vi "RamCtrl_Traj_UpdDiagGlobals.vi"(9 "outRAMSETE (SI)":T1 {"poseError"."ROTATION"."SIN" format="%13.4f"; "poseError"."ROTATION"."COS" format="%13.4f"; "poseError"."ROTATION"."VALUE" format="%13.4f"; "poseError"."TRANSLATION"."Y" format="%14.3f"; "poseError"."TRANSLATION"."X" format="%14.3f"; "poseTolerance"."ROTATION"."SIN" format="%13.4f"; "poseTolerance"."ROTATION"."COS" format="%13.4f"; "poseTolerance"."ROTATION"."VALUE" format="%13.4f"; "poseTolerance"."TRANSLATION"."Y" format="%14.3f"; "poseTolerance"."TRANSLATION"."X" format="%14.3f"; "Zeta" format="%12.3f"; "B" format="%12.3f"}, 10 "AtReference":bool, 11 "OutputTRAJ_STATE (SI)":T5 {"POSE"."ROTATION"."SIN" format="%13.4f"; "POSE"."ROTATION"."COS" format="%13.4f"; "POSE"."ROTATION"."VALUE" format="%13.4f"; "POSE"."TRANSLATION"."Y" format="%14.3f"; "POSE"."TRANSLATION"."X" format="%14.3f"}) -> ()   [LabVIEW 2019]
uses:
  <vilib>/Rock Robotics/WPI/ThirdParty/JAS_Junk/TrajLib/TypeDef/TRAJ_STATE.ctl
  <vilib>/Rock Robotics/WPI/ThirdParty/JAS_Junk/TrajLib/TypeDef/POSE2D.ctl
  <vilib>/Rock Robotics/WPI/ThirdParty/JAS_Junk/TrajLib/TypeDef/TRANSLATION2D.ctl
  <vilib>/Rock Robotics/WPI/ThirdParty/JAS_Junk/TrajLib/TypeDef/ROTATION2D.ctl
  <vilib>/Rock Robotics/WPI/ThirdParty/JAS_Junk/TrajLib/TypeDef/RAMSETE.ctl
  <vilib>/Rock Robotics/WPI/ThirdParty/JAS_Junk/TrajLib/Conv_Meters_Feet.vi
  <vilib>/Rock Robotics/WPI/ThirdParty/JAS_Junk/TrajLib/Conv_Radians_Deg.vi
  RamCtrl_Traj_Globals.vi
  <vilib>/Rock Robotics/WPI/ThirdParty/JAS_Junk/TrajLib/Trajectory_Library.lvlib
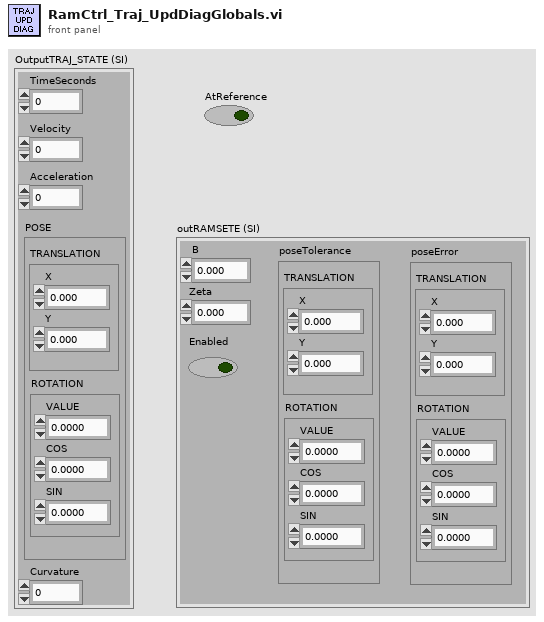
[diagram p1: front panel]
types:
  T1 = typedef "Trajectory_Library.lvlib/RAMSETE.ctl" = cluster{"B":dbl, "Zeta":dbl, "poseTolerance":T2, "poseError":T2, "Enabled":bool}
  T2 = typedef "Trajectory_Library.lvlib/POSE2D.ctl" = cluster{"TRANSLATION":T3, "ROTATION":T4}
  T3 = typedef "Trajectory_Library.lvlib/TRANSLATION2D.ctl" = cluster{"X":dbl, "Y":dbl}
  T4 = typedef "Trajectory_Library.lvlib/ROTATION2D.ctl" = cluster{"VALUE":dbl, "COS":dbl, "SIN":dbl}
  T5 = typedef "Trajectory_Library.lvlib/TRAJ_STATE.ctl" = cluster{"TimeSeconds":dbl, "Velocity":dbl, "Acceleration":dbl, "POSE":T2, "Curvature":dbl}
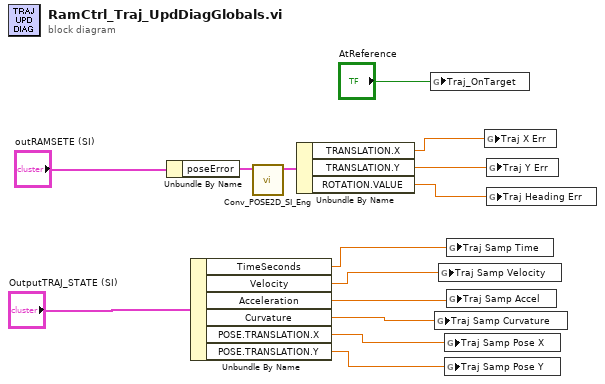
[diagram p0: block diagram]
diagram:
  n1 = Unbundle By Name("outRAMSETE (SI)") -> ("poseError"=w12:T2)
  n2 = Unbundle By Name("OutputTRAJ_STATE (SI)") -> ("TimeSeconds"=w6:dbl, "Velocity"=w5:dbl, "Acceleration"=w4:dbl, "Curvature"=w3:dbl, "POSE.TRANSLATION.X"=w2:dbl, "POSE.TRANSLATION.Y"=w1:dbl)
  n3 = call <vilib>:"Conv_POSE2D_SI_Eng.vi"("Err Pose in SI"=w12) -> ("Err Pose out ENG"=w13:T2)  [unwired: 10 in]
  n4 = Unbundle By Name(w13) -> ("TRANSLATION.X"=w9:dbl, "TRANSLATION.Y"=w8:dbl, "ROTATION.VALUE"=w7:dbl)
  n5 = global write "RamCtrl_Traj_Globals.vi" "Traj_OnTarget"("AtReference") -> ()
  n6 = global write "RamCtrl_Traj_Globals.vi" "Traj Samp Curvature"(w3) -> ()
  n7 = global write "RamCtrl_Traj_Globals.vi" "Traj Samp Velocity"(w5) -> ()
  n8 = global write "RamCtrl_Traj_Globals.vi" "Traj Samp Pose X"(w2) -> ()
  n9 = global write "RamCtrl_Traj_Globals.vi" "Traj Samp Pose Y"(w1) -> ()
  n10 = global write "RamCtrl_Traj_Globals.vi" "Traj Samp Time"(w6) -> ()
  n11 = global write "RamCtrl_Traj_Globals.vi" "Traj Samp Accel"(w4) -> ()
  n12 = global write "RamCtrl_Traj_Globals.vi" "Traj X Err"(w9) -> ()
  n13 = global write "RamCtrl_Traj_Globals.vi" "Traj Y Err"(w8) -> ()
  n14 = global write "RamCtrl_Traj_Globals.vi" "Traj Heading Err"(w7) -> ()
